vi "clone.vi"(0 "Numeric":dbl, 11 "Error in":errorcluster) -> (4 "Numeric Out":dbl, 6 "VI Clone Name":string, 8 "reference out":refnum<vi>, 15 "Error out":errorcluster)   [LabVIEW 2020, in "Reentrancy.lvlib"]
uses:
  Reentrancy.lvlib
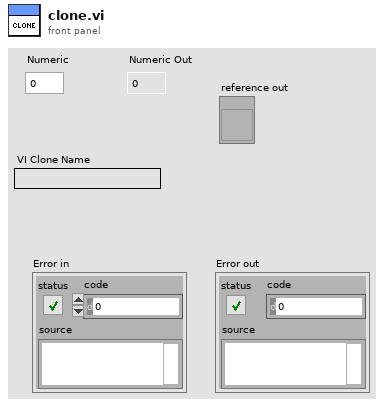
[diagram p1: front panel]
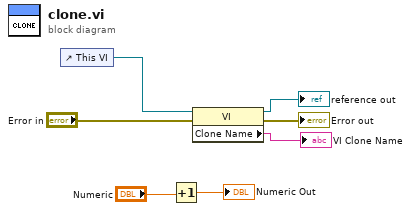
[diagram p0: block diagram]
diagram:
  n1 = control-ref of="This VI"() -> (w7:refnum<vi>)
  n2 = Increment(x="Numeric") -> (x+1=→"Numeric Out":dbl)
  n3 = property class="VI"(reference=w7, error in="Error in") -> (reference out=→"reference out":refnum<vi>, error out=→"Error out":errorcluster, "Clone Name"=→"VI Clone Name":string)
